vi "Add Plugin.vi"(8 "error in (no error)":errorcluster, 9 "Plugin":refnum<class "Plugin.lvclass">, 10 "parent tag":string, 11 "Application Data In":T1) -> (0 "error out":errorcluster, 2 "new item tag":string, 3 "Application Data In":T1)   [LabVIEW 2017, in "DSF Core.lvlib"]
uses:
  DSF Core.lvlib
  Main VI/Application Data.ctl
  <vilib>/NI/Memory Manager/Classes/Pointer/Pointer.lvclass
  Classes/Framework/Framework.lvclass
  Buffer Reader/Buffer Data.ctl
  Classes/Buffer/Buffer.lvclass
  Classes/Transfer Group Status/Transfer Group Status.lvclass
  Classes/Plugin/Plugin.lvclass
  Classes/Plugin/Plugin.lvclass/Plugin.ctl
  ID to Tree Items/Tree Item Type.ctl
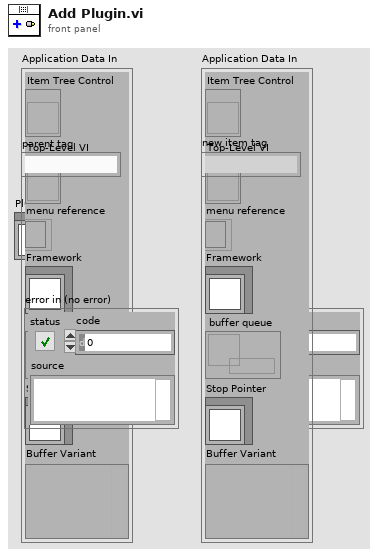
[diagram p1: front panel]
types:
  T1 = typedef "DSF Core.lvlib/Application Data.ctl" = cluster{"Item Tree Control":refnum<vi>, "Top-Level VI":refnum<vi>, "menu reference":refnum<k9>, "Framework":refnum<class "Framework.lvclass">, "buffer queue":refnum<queue>, "Stop Pointer":refnum<class "Pointer.lvclass">, "Buffer Variant":variant}
  T2 = typedef "DSF Core.lvlib/Tree Item Type.ctl" = enum16{"Framework", "Plugin Group", "Plugin", "Group", "Transfer", "Buffer", "Channel"}
  T3 = typedef "DSF Core.lvlib/Tree Item.ctl" = cluster{"Left Cell String":string, "Child Text":string[], "Child Tag":string, "Glyph Index":i32}
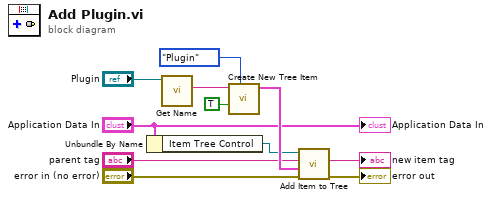
[diagram p0: block diagram]
diagram:
  n1 = Unbundle By Name("Application Data In") -> ("Item Tree Control"=w2:refnum<vi>)
  n2 = call "Get Name.vi"("Plugin in"="Plugin") -> ("name"=w9:string)  [unwired: 9 in, 1 out]
  n3 = call "Create New Tree Item.vi"("Item Type"=Tree_Item_Type."Plugin", "found?"=TRUE, "Left Cell String"=w9) -> ("Item"=w11:T3)  [unwired: 7 in, 1 out]
  n4 = call "Add Item to Tree.vi"("error in (no error)"="error in (no error)", "Item"=w11, "parent tag"="parent tag", "TreeControl in"=w2) -> ("error out"=→"error out":errorcluster, "new item tag"=→"new item tag":string)  [unwired: 5 in, 1 out]
  "Application Data In" <- "Application Data In"
